vi "3 Parallel Loops.vi"() -> ()   [LabVIEW 2014]
uses:
  <vilib>/Analysis/NI_AALBase.lvlib
panel:
  out "Analysis LED":bool
  in  "Stop Button":bool
  out "Histogram":dynamicdata(graph)
  out "STD":dbl(knob) scale=0.0..100.0
  out "Mean":dbl(knob) scale=0.0..100.0
  out "Thermometer":dbl(slide) scale=0.0..100.0
  out "Waveform Chart":dbl(graph)
  in  "Enable Analysis":bool
  in  "Temp":dbl(knob) scale=0.0..100.0
  # "Parallel Loops (Pahse 2)"
  # "Temperature"
  # "Temperature Log"
  # "Statistics"
  # "Statistics"
  # "Analysis \nStatus"
  # "Exit Program"
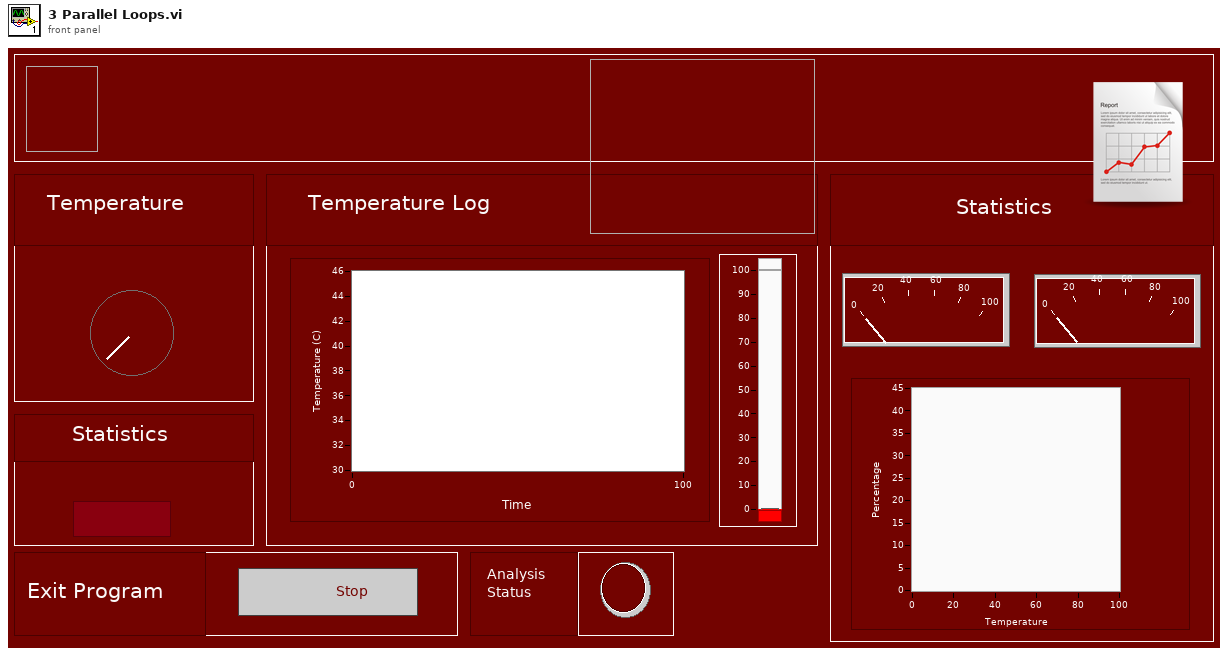
[diagram p1: front panel]
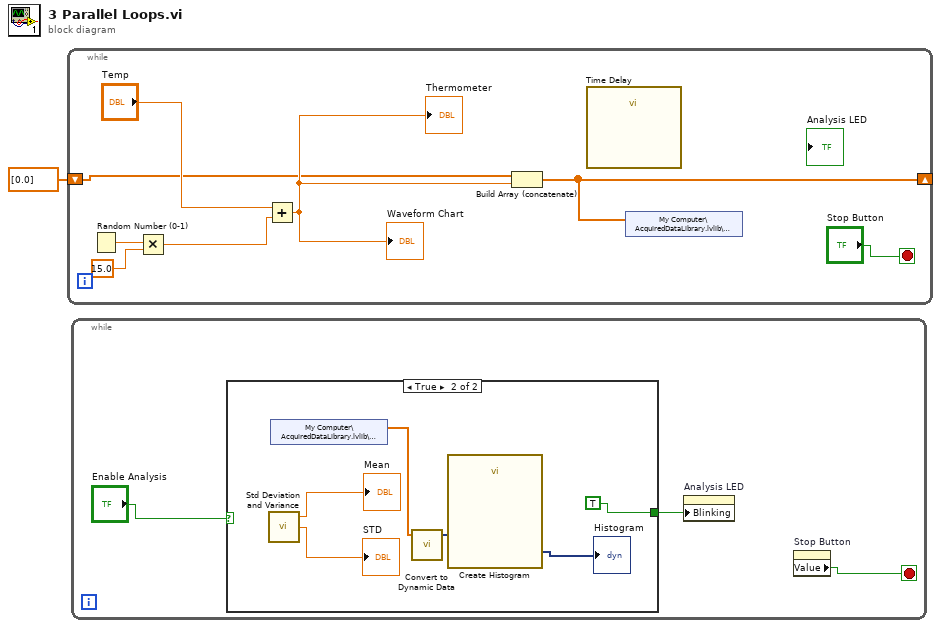
[diagram p0: block diagram]
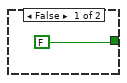
[diagram p2: hidden frame]
diagram:
  n1 = while {
    shift-right: [w2] -> _
    shift-left: dbl[] [0.0] -> [w3]
    stop <- "Stop Button" stop-if-true
    n2 = Random Number (0-1)() -> (number: 0 to 1=w8:dbl)
    n3 = Multiply(x=w8, y=15.0) -> (x*y=w6:dbl)
    n4 = Add(x="Temp", y=w6) -> (x+y=w5:dbl)
    "Waveform Chart" <- w5
    "Thermometer" <- w5
    n5 = Build Array (concatenate)(w3, w5) -> (w2:dbl[])
    n6 = call "Time Delay"() -> ()  [unwired: 11 in, 1 out]
    n7 = shared-variable "My Computer\\AcquiredDataLibrary.lvlib\\AcquiredData"(w2) -> ()  [unwired: 1 in, 1 out]
  }
  n8 = while {
    stop <- w12 stop-if-true
    n9 = case shown="True" "Enable Analysis" {
      tunnel: [FALSE TRUE] -> w11
      frame False {
      }
      frame True {
        n10 = call <vilib>:"Std Deviation and Variance.vi"() -> ("mean"=→"Mean":dbl, "standard deviation"=→"STD":dbl)  [unwired: 2 in, 1 out]
        n11 = shared-variable "My Computer\\AcquiredDataLibrary.lvlib\\AcquiredData"() -> (w14:dbl[])  [unwired: 1 in, 1 out]
        n12 = call "Convert to Dynamic Data"("Array"=w14) -> ("Dynamic Data Type"=w17:dynamicdata)  [unwired: 3 in]
        n13 = call "Create Histogram"("Signal"=w17) -> ("Histogram"=→"Histogram":dynamicdata)  [unwired: 9 in, 1 out]
      }
    }
    n14 = property on="Analysis LED" class="Bool (strict)"("Blinking"=w11) -> ()  [unwired: 2 in, 2 out]
    n15 = property on="Stop Button" class="Bool (strict)"() -> ("Value"=w12:bool)  [unwired: 2 in, 2 out]
  }
